vi "Proyecto Puntos extra RGB y Sensor infrarojo.vi"() -> ()   [LabVIEW 2026]
uses:
  <vilib>/MakerHub/LINX/Public/Peripherals/Digital/Digital Write 1 Chan.vi
  <vilib>/MakerHub/LINX/Public/Peripherals/Digital/Digital Write N Chans.vi
  <vilib>/MakerHub/LINX/Private/Local IO/LinxDigitalWrite.vi
  <vilib>/MakerHub/LINX/Public/Utilities/Check Channel.vi
  <vilib>/MakerHub/LINX/Private/Utilties/Generate Error.vi
  <vilib>/MakerHub/LINX/Public/Utilities/Open Serial.vi
  <vilib>/MakerHub/LINX/LMH-LINX.lvlib
panel:
  in  "Serial Port":refnum<visa-resource-name>="N/A"
  out "ESTADO DE LA ALARMA 2":string
  in  "CONFIGURACION":bool
  in  "ALARMAA":bool
  in  "stop":bool
  out "ESTADO":bool
  out "ESTADO DE LA ALARMA":string
  out "ALARMA":bool
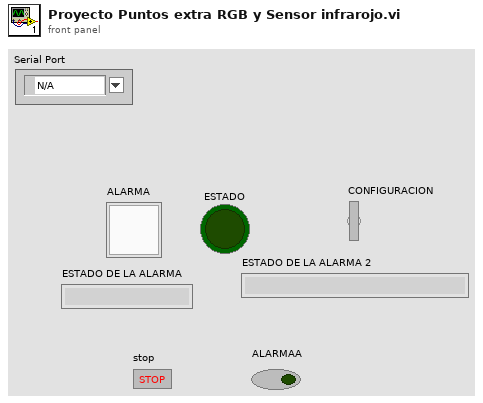
[diagram p1: front panel]
types:
  T1 = typedef "LMH-LINX.lvlib/LINX Ref.ctl" = cluster{"IO":T2, "Interface":T3, "LINX Device Config":T4}
  T2 = typedef "LMH-LINX.lvlib/Platform.ctl" = enum16{"Remote", "Local"}
  T3 = typedef "LMH-LINX.lvlib/Interface.ctl" = enum16{"Serial", "TCP"}
  T4 = typedef "LMH-LINX.lvlib/Device.lvlib/LINX Device Config.ctl" = cluster{"Interface":T3, "COM Port":refnum<visa-resource-name>, "TCP Configuration":T5, "Device Family":u8, "Device ID":u8, "Device Name":string, "TCP Ref":refnum<k5>, "Channels":T6}
  T5 = typedef "LMH-LINX.lvlib/Device.lvlib/TCP Config.ctl" = cluster{"IP Address":string, "Port":u16}
  T6 = typedef "LMH-LINX.lvlib/Channels.ctl" = cluster{"DI":u8[], "DO":u8[], "AI":u8[], "AO":u8[], "PWM":u8[], "QE":u8[], "UART":u8[], "I2C 2":u8[], "SPI":u8[], "CAN":u8[], "Servo":u8[], "AI Ref (V)":dbl, "AI Resolution (Bits)":u8, "AO Ref (V)":dbl, "AO Resolution (Bits)":u8}
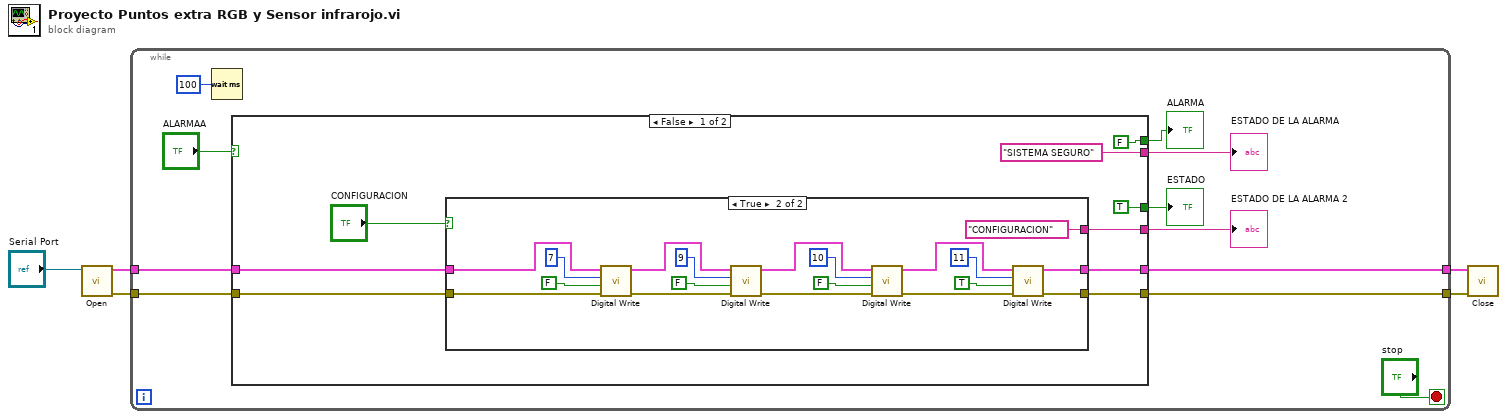
[diagram p0: block diagram]
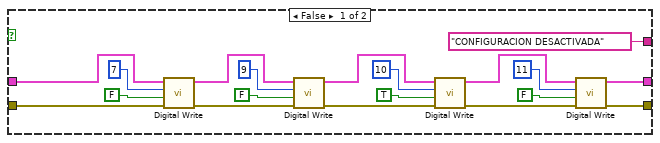
[diagram p2: hidden frame]
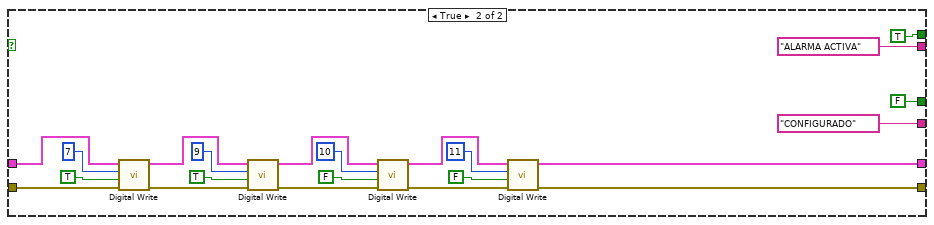
[diagram p3: hidden frame]
diagram:
  n1 = call-poly <vilib>:"Open.vi"("Serial Port"="Serial Port") -> ("Error Out"=w4:errorcluster, "LINX Resource"=w5:T1)  [unwired: 8 in, 1 out]
  n2 = while {
    tunnel: w5 -> [w12]
    tunnel: w4 -> [w13]
    tunnel: [w10] -> w3
    tunnel: [w11] -> w2
    stop <- "stop" stop-if-true
    n3 = Wait (ms)(milliseconds to wait=u32 100) -> ()  [unwired: 1 out]
    n4 = case shown="False" "ALARMAA" {
      tunnel: ["SISTEMA SEGURO" "ALARMA ACTIVA"] -> w14
      tunnel: [FALSE TRUE] -> w9
      tunnel: w13 -> [w21 w84]
      tunnel: w12 -> [w20 w82]
      tunnel: [w19 w81] -> w11
      tunnel: [w18 w80] -> w10
      tunnel: [TRUE FALSE] -> w8
      tunnel: [w17 "CONFIGURADO"] -> w6
      frame False {
        n5 = case shown="True" "CONFIGURACION" {
          tunnel: w21 -> [w44 w46]
          tunnel: w20 -> [w42 w47]
          tunnel: [w41 w52] -> w19
          tunnel: [w40 w53] -> w18
          tunnel: ["CONFIGURACION DESACTIVADA" "CONFIGURACION"] -> w17
          frame False {
            n6 = call-poly <vilib>:"Digital Write.vi"("Error In"=w44, "Output Value"=FALSE, "DO Channel"=u8 7, "LINX Resource"=w42) -> ("Error Out"=w38:errorcluster, "LINX Resource"=w39:T1)  [unwired: 6 in]
            n7 = call-poly <vilib>:"Digital Write.vi"("Error In"=w38, "Output Value"=FALSE, "DO Channel"=u8 9, "LINX Resource"=w39) -> ("Error Out"=w36:errorcluster, "LINX Resource"=w37:T1)  [unwired: 6 in]
            n8 = call-poly <vilib>:"Digital Write.vi"("Error In"=w36, "Output Value"=TRUE, "DO Channel"=u8 10, "LINX Resource"=w37) -> ("Error Out"=w34:errorcluster, "LINX Resource"=w35:T1)  [unwired: 6 in]
            n9 = call-poly <vilib>:"Digital Write.vi"("Error In"=w34, "Output Value"=FALSE, "DO Channel"=u8 11, "LINX Resource"=w35) -> ("Error Out"=w41:errorcluster, "LINX Resource"=w40:T1)  [unwired: 6 in]
          }
          frame True {
            n10 = call-poly <vilib>:"Digital Write.vi"("Error In"=w46, "Output Value"=FALSE, "DO Channel"=u8 7, "LINX Resource"=w47) -> ("Error Out"=w48:errorcluster, "LINX Resource"=w49:T1)  [unwired: 6 in]
            n11 = call-poly <vilib>:"Digital Write.vi"("Error In"=w48, "Output Value"=FALSE, "DO Channel"=u8 9, "LINX Resource"=w49) -> ("Error Out"=w50:errorcluster, "LINX Resource"=w55:T1)  [unwired: 6 in]
            n12 = call-poly <vilib>:"Digital Write.vi"("Error In"=w50, "Output Value"=FALSE, "DO Channel"=u8 10, "LINX Resource"=w55) -> ("Error Out"=w51:errorcluster, "LINX Resource"=w54:T1)  [unwired: 6 in]
            n13 = call-poly <vilib>:"Digital Write.vi"("Error In"=w51, "Output Value"=TRUE, "DO Channel"=u8 11, "LINX Resource"=w54) -> ("Error Out"=w52:errorcluster, "LINX Resource"=w53:T1)  [unwired: 6 in]
          }
        }
      }
      frame True {
        n14 = call-poly <vilib>:"Digital Write.vi"("Error In"=w84, "Output Value"=TRUE, "DO Channel"=u8 7, "LINX Resource"=w82) -> ("Error Out"=w74:errorcluster, "LINX Resource"=w79:T1)  [unwired: 6 in]
        n15 = call-poly <vilib>:"Digital Write.vi"("Error In"=w74, "Output Value"=TRUE, "DO Channel"=u8 9, "LINX Resource"=w79) -> ("Error Out"=w73:errorcluster, "LINX Resource"=w78:T1)  [unwired: 6 in]
        n16 = call-poly <vilib>:"Digital Write.vi"("Error In"=w73, "Output Value"=FALSE, "DO Channel"=u8 10, "LINX Resource"=w78) -> ("Error Out"=w72:errorcluster, "LINX Resource"=w77:T1)  [unwired: 6 in]
        n17 = call-poly <vilib>:"Digital Write.vi"("Error In"=w72, "Output Value"=FALSE, "DO Channel"=u8 11, "LINX Resource"=w77) -> ("Error Out"=w81:errorcluster, "LINX Resource"=w80:T1)  [unwired: 6 in]
      }
    }
    "ALARMA" <- w9
    "ESTADO DE LA ALARMA" <- w14
    "ESTADO" <- w8
    "ESTADO DE LA ALARMA 2" <- w6
  }
  n18 = call <vilib>:"Close.vi"("Error In"=w2, "LINX Resource"=w3) -> ()  [unwired: 9 in, 1 out]
